vi "3Dplotter.vi"(11 "vectorFile1":path) -> ()   [LabVIEW 2022 SP3]
uses:
  3-Dobject.ctl
  Anemometry/Utilities/EnQMH/EnQcmd.ctl
  <vilib>/Analysis/Matrix/Datatypes/RealMatrix.ctl
  3DplotterData.ctl
  vectorDef.ctl
  coordSys.ctl
  <vilib>/Utility/miscctls.llb/LVRGBAColorTypeDef.ctl
  <vilib>/Utility/miscctls.llb/LV3DPointTypeDef.ctl
  <vilib>/Analysis/baseanly.llb/Real A x B.vi
  <vilib>/Analysis/baseanly.llb/Real Dot Product.vi
  6d968bff-314f-d647-9bf6-e40cfc3952a7.vi
  08ae1a81-02f0-e744-b827-f8e6f0f1c480.vi
  4d4a6871-819a-da47-9cf5-1746fbad62e0.vi
  676242ff-a6cf-3e4f-a0ed-2fc44f2a90a5.vi
  <vilib>/Utility/error.llb/Trim Whitespace One-Sided.vi
  Anemometry/Utilities/EnQMH/EnQmsg.vi
  Anemometry/Utilities/EnQMH/EnQmsgs.vi
  <vilib>/Analysis/baseanly.llb/Real Inverse Matrix.vi
  <vilib>/picture/3D Picture Control/Object/Create Object (name).vi
  <vilib>/picture/3D Picture Control/Object/Add Object (reference).vi
  <vilib>/Comparison/Less/Less Functor/Less Functor.lvclass
  <vilib>/picture/3D Picture Control/Helpers/Apply Texture (no reference).vi
  <vilib>/picture/3D Picture Control/NI_3D Picture Control.lvlib
  <vilib>/Analysis/NI_AALBase.lvlib
  <vilib>/Analysis/Matrix/NI_Matrix.lvlib
panel:
  in  "Tab Control":T1(tab)
  in  "view":i32(slide) min=-1 max=1 step=1
  in  "exportSetup":bool
  in  "importSetup":bool
  in  "Wind Direction Selector":string(combo)
  in  "vectorFile2":path
  in  "Vector Scale":dbl(slide)=100.0 scale=0.2..200.0
  out "Color Ramp":dbl(ramp)
  in  "geometryScale":dbl(slide)=1.0 min=0.1 max=50.0 step=1.0 scale=0.1..50.0 scale format="%#_3g"
  in  "geometry":T2[](array[typedef])
  in  "geometrydZ":dbl(slide) scale=-20.0..20.0
  in  "rampOverride":bool
  in  "rampMax":dbl
  in  "rampMin":dbl
  in  "colourRampClip":dbl min=0.0 max=10.0 step=0.1 format="%#_g%%"
  in  "windrosePath":path
  in  "windrosedXdYdZ":cluster{"dX":dbl, "dY":dbl, "dZ":dbl}
  in  "Apply Mode":T3(ring)=enum."With Modulation"
  in  "windroseScale":dbl(slide)=1.046728971962617 scale=0.5..2.0
  in  "axesColour":u32(colorbox)=16739840
  in  "axes":bool=TRUE
  out "degSymbol":string
  out "eventLoop":errorcluster
  out "stopDolly":bool
  out "actionLoop":errorcluster
  in  "clearVectors":bool
  out "3D Picture":refnum<vi>(3d-picture)
  out "camStandoff":dbl caption="Camera Distance" format="%#.0f"
  in  "camLocn":dbl[](array[numeric]) caption="Camera Location" format="%#.0f"
  in  "Stop":bool
  in  "depthClipping":cluster{sgl, sgl, sgl}(slide)={0.001, 10.0, 9.712047e-08} scale=10.0..0.001 scale format="%.0pm"
  in  "FoV":sgl(slide)=50.0 min=4 max=110 scale=80.0..4.0 scale format="%dº"
  in  "drive":sgl(slide) min=-0.05 max=0.05 scale=0.03..-0.03 scale format="%#.1f"
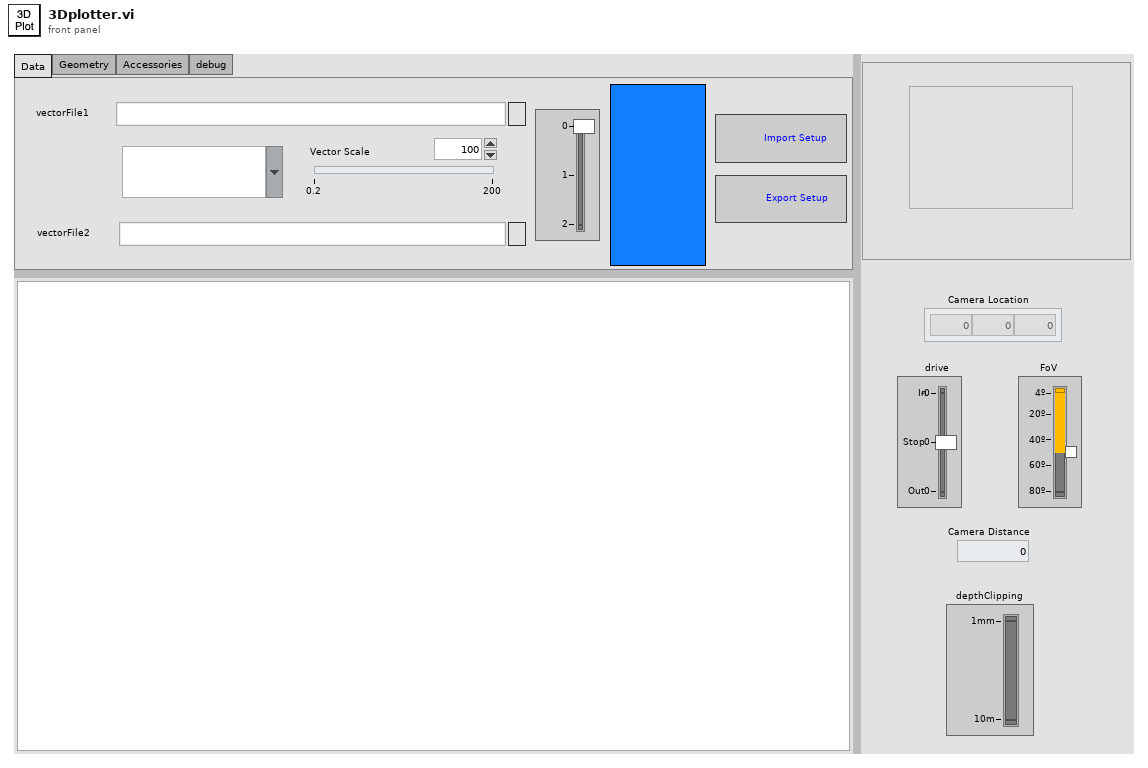
[diagram p1: front panel]
types:
  T1 = enum32{"Data", "Geometry", "Accessories", "debug"}
  T2 = typedef "3-Dobject.ctl" = cluster{"name":string, "path":path, "Colour":u32, "Visible":bool, "dZ":dbl}
  T3 = enum16{"As a Decal", "With Modulation", "With Blending", "As a replacement"}
  T4 = typedef "EnQcmd.ctl" = cluster{"message":string, "payload":variant}
  T5 = typedef "3DplotterData.ctl" = cluster{"mode":bool, "refWorld":refnum<vi>, "refAxes":refnum<vi>, "refWindrose":refnum<vi>, "refGeometry":refnum<vi>, "geometryRefs":refnum<vi>[], "refVectors":refnum<vi>, "refVecs1":refnum<vi>, "refVecs2":refnum<vi>, "vector1Info":T6, "file1scalar":dbl[], "vector2Info":T6, "file2scalar":dbl[], "colourRampVals":cluster{"value":dbl, "colour":u32}[]}
  T6 = typedef "vectorDef.ctl" = cluster{"pointID":string[], "XYZ-WD":dbl[][], "UVW-TI":dbl[][], "CoordSys":T7[]}
  T7 = typedef "coordSys.ctl" = enum16{"Tunnel", "Model"}
  T8 = enum16{"Inherit Value", "No Culling", "Cull Back Face", "Cull Front Face", "Cull Both Faces"}
  T9 = typedef "LVRGBAColorTypeDef.ctl" = cluster{"Red":sgl, "Green":sgl, "Blue":sgl, "Alpha":sgl}
  T10 = enum16{"Inherit Value", "Points", "Wireframe", "Polygons"}
  T11 = enum16{"Normal Bin", "Opaque Bin", "Transparent Bin"}
  T12 = typedef "imagedata.ctl" = cluster{"image type":i32, "image depth":i32, "image":u8[], "mask":u8[], "colors":u32[], "Rectangle":cluster{"left":i16, "top":i16, "right":i16, "bottom":i16}}
  T13 = typedef "Triangle.ctl" = cluster{"V0":sgl[], "V1":sgl[], "V2":sgl[], "E0":sgl[], "E1":sgl[], "E2":sgl[], "n^":sgl[], "nE0^":sgl[], "nE1^":sgl[], "nE2^":sgl[]}
  T14 = typedef "LV3DPointTypeDef.ctl" = cluster{"X":sgl, "Y":sgl, "Z":sgl}
  T15 = typedef "NI_Matrix.lvlib/RealMatrix.ctl" = dbl[][]
  T16 = enum32{"General", "Positive Definite", "Lower Triangular", "Upper Triangular"}
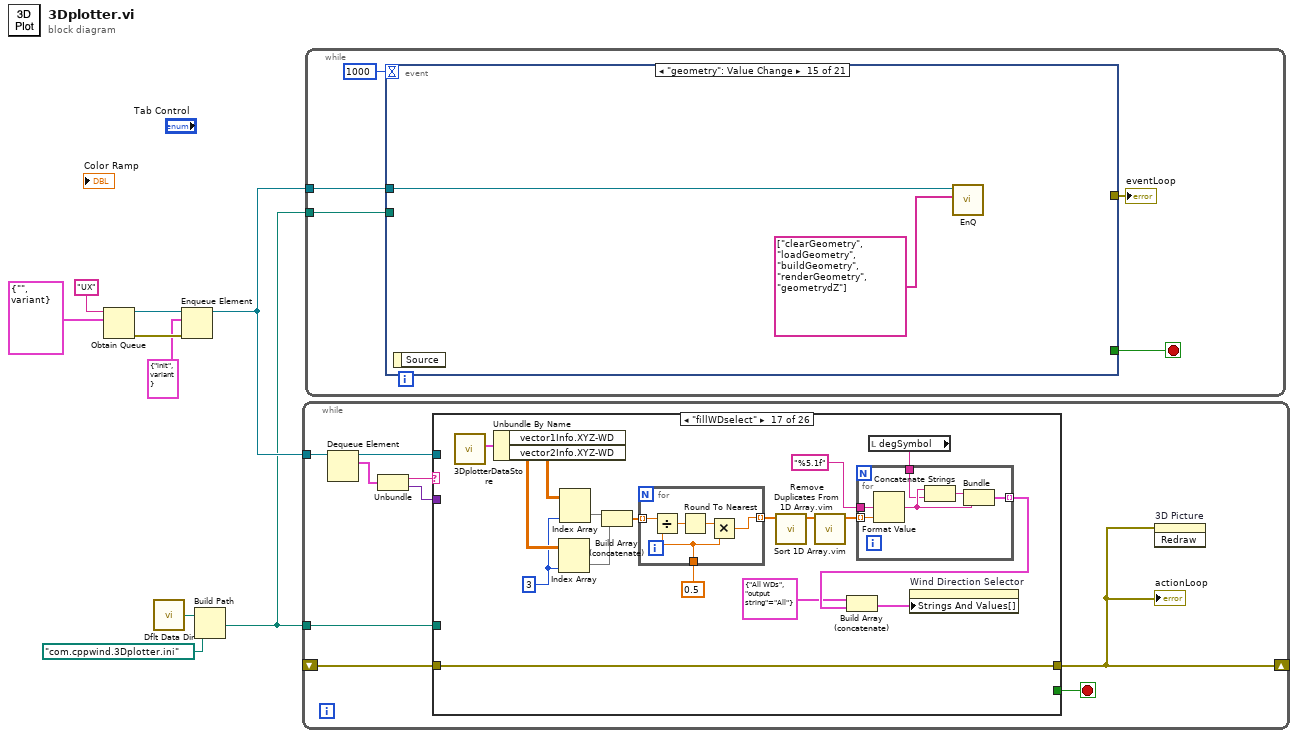
[diagram p0: block diagram]
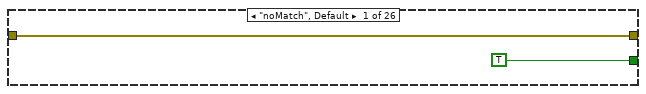
[diagram p2: hidden frame]
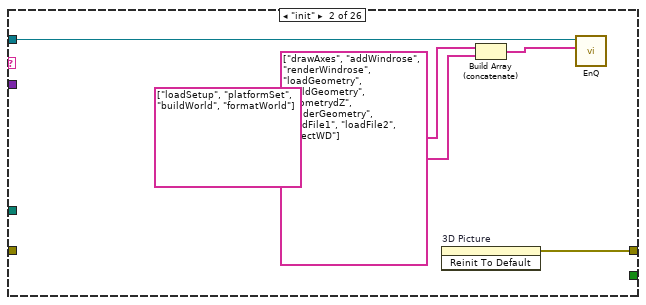
[diagram p3: hidden frame]
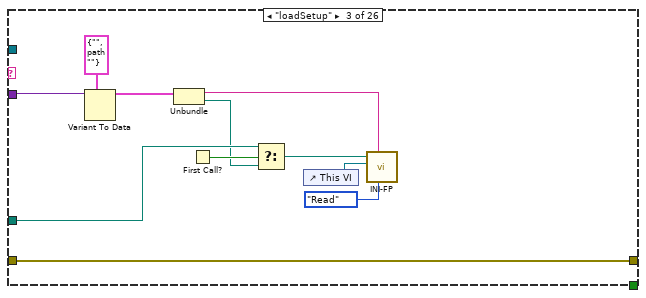
[diagram p4: hidden frame]
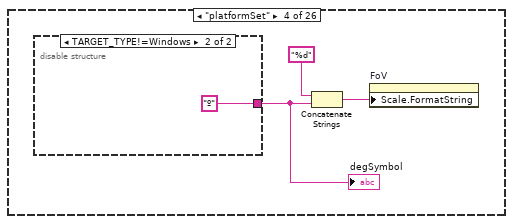
[diagram p5: hidden frame]
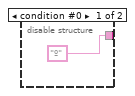
[diagram p6: hidden frame]
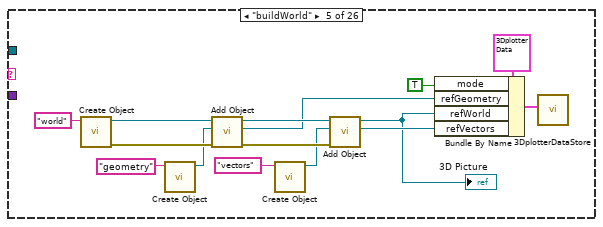
[diagram p7: hidden frame]
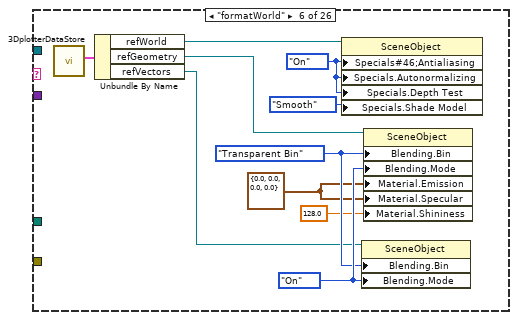
[diagram p8: hidden frame]
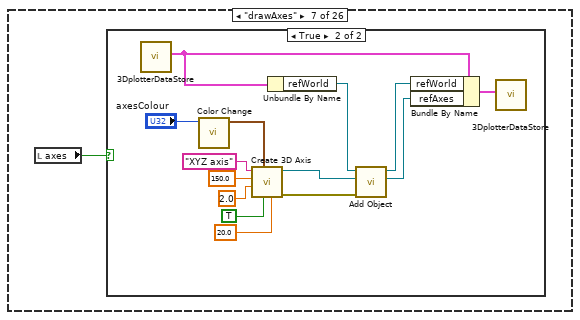
[diagram p9: hidden frame]
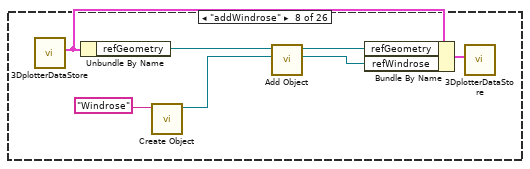
[diagram p11: hidden frame]
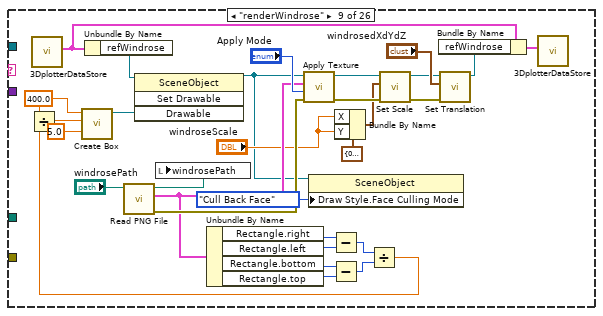
[diagram p12: hidden frame]
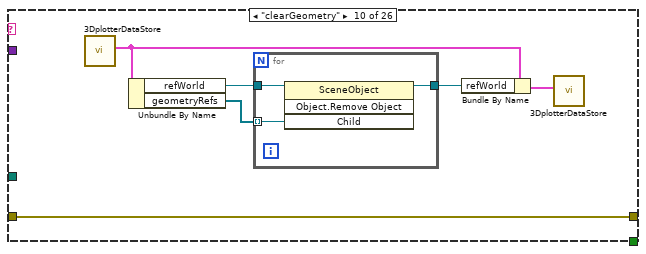
[diagram p13: hidden frame]
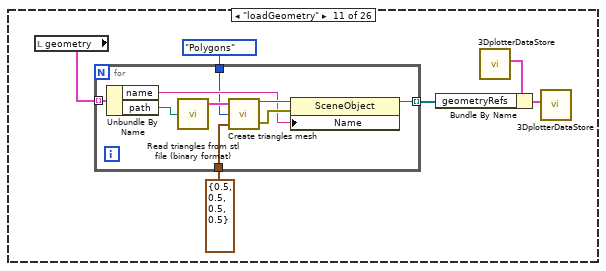
[diagram p14: hidden frame]
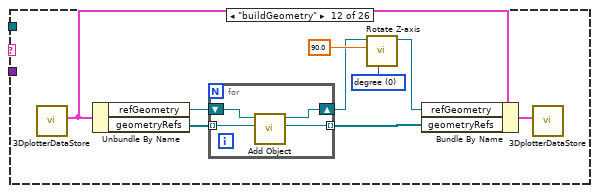
[diagram p15: hidden frame]
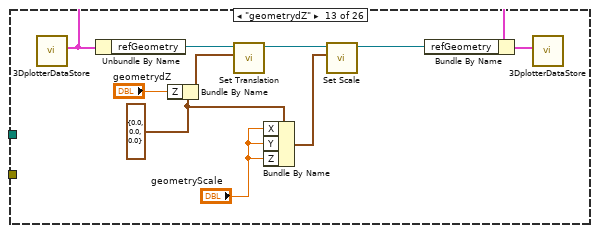
[diagram p16: hidden frame]
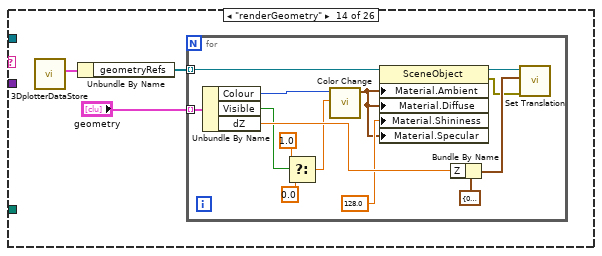
[diagram p17: hidden frame]
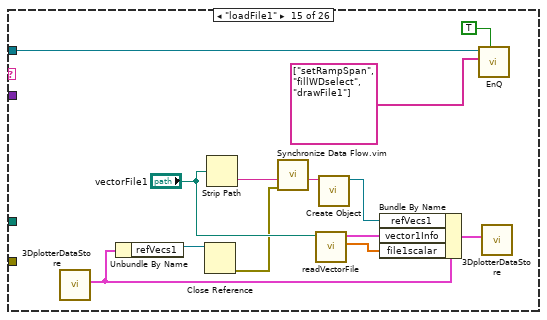
[diagram p18: hidden frame]
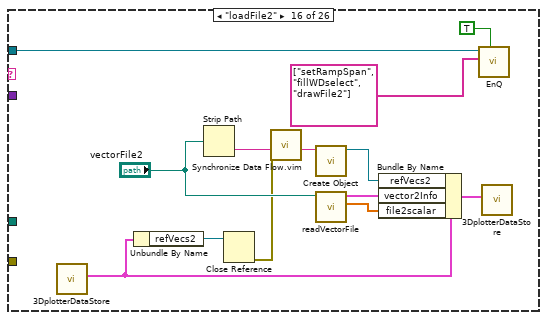
[diagram p19: hidden frame]
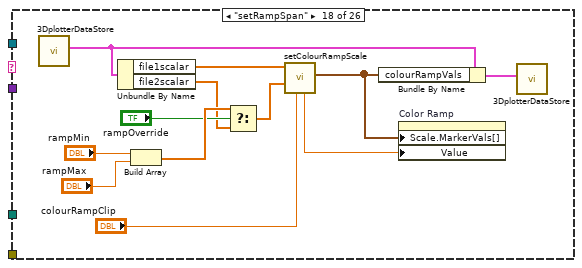
[diagram p20: hidden frame]
diagram:
  n1 = Obtain Queue(name (unnamed)="UX", element data type=T4 {"message"="", "payload"=variant} ("command")) -> (queue out=w5:refnum<queue>, error out=w9:errorcluster)  [unwired: 3 in, 1 out]
  n2 = call <vilib>:"Dflt Data Dir.vi"() -> ("App:Default Data Directory"=w3:path)
  n3 = Enqueue Element(queue=w5, element=T4 {"message"="init", "payload"=variant}, error in (no error)=w9) -> (queue out=w4:refnum<queue>)  [unwired: 1 in, 2 out]
  n4 = Build Path(base path=w3, name or relative path=path "com.cppwind.3Dplotter.ini") -> (appended path=w1:path)
  n5 = while {
    tunnel: w4 -> [w18]
    shift-right: [w10] -> _
    shift-left: _ -> [w13]
    tunnel: w1 -> [w11]
    stop <- w15 stop-if-true
    n6 = Dequeue Element(queue=w18) -> (queue out=w14:refnum<queue>, element=w17:T4)  [unwired: 2 in, 2 out]
    n7 = Unbundle(w17) -> ("message"=w12:string, "payload"=w16:variant)
    n8 = case shown="\"fillWDselect\"" w12 {
      tunnel: w16 -> [_ _ w31 _ _ _ _ _ _ _ _ _ _ _ _ _ _ _ _ _ _ _ _ _ w332 _]
      tunnel: [TRUE _ _ _ _ _ _ _ _ _ _ _ _ _ _ _ _ _ _ _ _ _ _ _ _ TRUE] -> w15
      tunnel: w14 -> [_ w24 _ _ _ _ _ _ _ _ _ _ _ _ w192 w205 _ _ _ _ _ _ _ _ _ _]
      tunnel: [w19 w25 w36 _ _ _ _ _ _ w124 _ _ _ _ _ _ w225 _ _ _ _ _ _ _ w327 _] -> w10
      tunnel: w13 -> [w19 _ w36 _ _ _ _ _ _ w124 _ _ _ _ _ _ w225 _ _ _ _ _ _ _ _ _]
      tunnel: w11 -> [_ _ w28 _ _ _ _ _ _ _ _ _ _ _ _ _ _ _ _ _ _ _ _ _ _ _]
      frame "noMatch", Default {
      }
      frame "init" {
        n9 = invoke on="3D Picture" class="SceneGraphDisp (strict)" method="Reinit To Default"() -> (error out=w25:errorcluster)  [unwired: 3 in, 2 out]
        n10 = Build Array (concatenate)(string[] ["loadSetup", "platformSet", "buildWorld", "formatWorld"] ("messages"), string[] ["drawAxes", "addWindrose", "renderWindrose", "loadGeometry", "buildGeometry", "geometrydZ", "renderGeometry", "loadFile1", "loadFile2", "selectWD"] ("messages")) -> (w21:string[])
        n11 = call-poly "EnQ.vi"("messages"=w21, "EnQin"=w24) -> ()  [unwired: 7 in, 3 out]
      }
      frame "loadSetup" {
        n12 = Variant To Data(type=cluster{string, "appended path":path} {"", "appended path"=path ""} ("output cluster"), Variant=w31) -> (data=w33:cluster{string, "appended path":path})  [unwired: 1 in, 1 out]
        n13 = Unbundle(w33) -> (w30:string, "appended path"=w27:path)
        n14 = First Call?() -> (First Call?: T/F=w29:bool)
        n15 = Select(t=w28, s=w29, f=w27) -> (s? t:f=w26:path)
        n16 = control-ref of="This VI"() -> (w35:refnum<vi>)
        n17 = call "INI-FP.vi"("Mode"=enum16{"Read", "Write"}."Read", "prompt"=w30, "VIreference"=w35, "INIfilepathIn"=w26) -> ()  [unwired: 6 in, 2 out]
      }
      frame "platformSet" {
        n18 = disable-structure shown="TARGET_TYPE!=Windows" {
          disable-tunnel: ["º" ("Scale.Format String") "º" ("Scale.Format String")] -> w37
          frame condition #0 {
          }
          frame condition #1 (active) {
          }
        }
        "degSymbol" <- w37
        n19 = Concatenate Strings("%d" ("Scale.Format String"), w37) -> (w39:string)
        n20 = property on="FoV" class="Slide (strict)"("Scale.FormatString"=w39) -> ()  [unwired: 2 in, 2 out]
      }
      frame "buildWorld" {
        n21 = call-poly <vilib>:"Create Object.vi"("Name"="world") -> ("error out"=w48:errorcluster, "Scene:New Object"=w50:refnum<vi>)  [unwired: 9 in]
        n22 = call-poly <vilib>:"Create Object.vi"("Name"="geometry") -> ("Scene:New Object"=w44:refnum<vi>)  [unwired: 9 in, 1 out]
        n23 = call-poly <vilib>:"Add Object.vi"("error in (no error)"=w48, "New Object In"=w44, "Scene Object In"=w50) -> ("error out"=w47:errorcluster, "New Object Out"=w46:refnum<vi>, "Scene Object Out"=w49:refnum<vi>)  [unwired: 6 in]
        n24 = call-poly <vilib>:"Create Object.vi"("Name"="vectors") -> ("Scene:New Object"=w43:refnum<vi>)  [unwired: 9 in, 1 out]
        n25 = call-poly <vilib>:"Add Object.vi"("error in (no error)"=w47, "New Object In"=w43, "Scene Object In"=w49) -> ("New Object Out"=w45:refnum<vi>, "Scene Object Out"=w42:refnum<vi>)  [unwired: 6 in, 1 out]
        "3D Picture" <- w42
        n26 = Bundle By Name(cluster=T5 {"mode"=FALSE, "refWorld"=refnum, "refAxes"=refnum, "refWindrose"=refnum, "refGeometry"=refnum, "geometryRefs"=[], "refVectors"=refnum, "refVecs1"=refnum, "refVecs2"=refnum, "vector1Info"={"pointID"=[], "XYZ-WD"=[], "UVW-TI"=[], "CoordSys"=[]}, "file1scalar"=[], "vector2Info"={"pointID"=[], "XYZ-WD"=[], "UVW-TI"=[], "CoordSys"=[]}, "file2scalar"=[], "colourRampVals"=[]} ("3DplotterDataIn"), "mode"=TRUE, "refGeometry"=w46, "refWorld"=w42, "refVectors"=w45) -> (w53:T5)
        n27 = call "3DplotterDataStore.vi"("3DplotterDataIn"=w53) -> ()  [unwired: 10 in, 1 out]
      }
      frame "formatWorld" {
        w62 = enum16{"Inherit Value", "Off", "On"}."On" ("Specials:Anti-aliasing")
        w64 = T9 {"Red"=0.0, "Green"=0.0, "Blue"=0.0, "Alpha"=0.0} ("Material:Emission")
        w66 = enum16{"Inherit Value", "Off", "On"}."On" ("Blending:Mode")
        w65 = T11."Transparent Bin" ("Blending:Bin")
        n28 = call "3DplotterDataStore.vi"() -> ("3DplotterDataOut"=w60:T5)  [unwired: 11 in]
        n29 = Unbundle By Name(w60) -> ("refWorld"=w59:refnum<vi>, "refGeometry"=w58:refnum<vi>, "refVectors"=w57:refnum<vi>)
        n30 = property class="SceneObject"(reference=w59, "Specials#46;Antialiasing"=w62, "Specials.Autonormalizing"=w62, "Specials.Depth Test"=w62, "Specials.Shade Model"=enum16{"Inherit Value", "Flat", "Smooth"}."Smooth" ("Specials:Shade Model")) -> ()  [unwired: 1 in, 2 out]
        n31 = property class="SceneObject"(reference=w57, "Blending.Bin"=w65, "Blending.Mode"=w66) -> ()  [unwired: 1 in, 2 out]
        n32 = property class="SceneObject"(reference=w58, "Blending.Bin"=w65, "Blending.Mode"=w66, "Material.Emission"=w64, "Material.Specular"=w64, "Material.Shininess"=sgl 128.0 ("Material:Shininess")) -> ()  [unwired: 1 in, 2 out]
      }
      frame "drawAxes" {
        n33 = local read "axes"() -> (w67:bool)
        n34 = case shown="True" w67 {
          frame False {
          }
          frame True {
            n35 = call "3DplotterDataStore.vi"() -> ("3DplotterDataOut"=w75:T5)  [unwired: 11 in]
            n36 = call <vilib>:"Color Change.vi"("Color"="axesColour") -> ("RGBA"=w69:cluster{"R":sgl, "G":sgl, "B":sgl, "A":sgl})  [unwired: 10 in]
            n37 = call <vilib>:"Create 3D Axis.vi"("Character Size"=sgl 20.0, "Axis label?"=TRUE, "Color"=w69, "Radius"=sgl 2.0, "Length"=sgl 150.0, "Name"="XYZ axis") -> ("error out"=w71:errorcluster, "New Object Refnum"=w73:refnum<vi>)  [unwired: 4 in]
            n38 = Unbundle By Name(w75) -> ("refWorld"=w74:refnum<vi>)
            n39 = call-poly <vilib>:"Add Object.vi"("error in (no error)"=w71, "New Object In"=w73, "Scene Object In"=w74) -> ("New Object Out"=w72:refnum<vi>, "Scene Object Out"=w70:refnum<vi>)  [unwired: 6 in, 1 out]
            n40 = Bundle By Name(cluster=w75, "refWorld"=w70, "refAxes"=w72) -> (w81:T5)
            n41 = call "3DplotterDataStore.vi"("3DplotterDataIn"=w81) -> ()  [unwired: 10 in, 1 out]
          }
        }
      }
      frame "addWindrose" {
        n42 = call "3DplotterDataStore.vi"() -> ("3DplotterDataOut"=w85:T5)  [unwired: 11 in]
        n43 = Unbundle By Name(w85) -> ("refGeometry"=w88:refnum<vi>)
        n44 = call-poly <vilib>:"Create Object.vi"("Name"="Windrose") -> ("Scene:New Object"=w82:refnum<vi>)  [unwired: 9 in, 1 out]
        n45 = call-poly <vilib>:"Add Object.vi"("New Object In"=w82, "Scene Object In"=w88) -> ("New Object Out"=w83:refnum<vi>, "Scene Object Out"=w84:refnum<vi>)  [unwired: 7 in, 1 out]
        n46 = Bundle By Name(cluster=w85, "refGeometry"=w84, "refWindrose"=w83) -> (w86:T5)
        n47 = call "3DplotterDataStore.vi"("3DplotterDataIn"=w86) -> ()  [unwired: 10 in, 1 out]
      }
      frame "renderWindrose" {
        w100 = sgl 400.0 ("Length X")
        n48 = call "3DplotterDataStore.vi"() -> ("3DplotterDataOut"=w112:T5)  [unwired: 11 in]
        n49 = Unbundle By Name(w112) -> ("refWindrose"=w111:refnum<vi>)
        n50 = call <vilib>:"Read PNG File.vi"("path to PNG file"="windrosePath") -> ("error out"=w116:errorcluster, "image data"=w109:T12, "path"=w89:path)  [unwired: 8 in]
        n51 = local write "windrosePath"(w89) -> ()
        n52 = Unbundle By Name(w109) -> ("Rectangle.right"=w108:i16, "Rectangle.left"=w107:i16, "Rectangle.bottom"=w106:i16, "Rectangle.top"=w105:i16)
        n53 = Subtract(x=w108, y=w107) -> (x-y=w104:i16)
        n54 = Subtract(x=w106, y=w105) -> (x-y=w103:i16)
        n55 = Bundle By Name(cluster=cluster{"X":sgl, "Y":sgl, "Z":sgl} {"X"=0.0, "Y"=0.0, "Z"=0.0} ("Scale"), "X"="windroseScale", "Y"="windroseScale") -> (w94:cluster{"X":sgl, "Y":sgl, "Z":sgl})
        n56 = Divide(x=w104, y=w103) -> (x/y=w102:dbl)
        n57 = Divide(x=w100, y=w102) -> (x/y=w101:dbl)
        n58 = call <vilib>:"Create Box.vi"("Length Z"=sgl 5.0, "Length Y"=w101, "Length X"=w100) -> ("New Box Refnum"=w110:refnum<vi>)  [unwired: 7 in, 1 out]
        n59 = invoke class="SceneObject" method="Set Drawable"(reference=w111, "Drawable"=w110) -> (reference out=w91:refnum<vi>)  [unwired: 2 in, 3 out]
        n60 = call-poly <vilib>:"Apply Texture.vi"("error in (no error)"=w116, "Apply Mode"="Apply Mode", "Image Data"=w109, "Scene Object In"=w91) -> ("error out"=w98:errorcluster, "Scene Object Out"=w99:refnum<vi>)  [unwired: 6 in]
        n61 = property class="SceneObject"(reference=w91, "Draw Style.Face Culling Mode"=T8."Cull Back Face" ("Draw Style:Face Culling Mode")) -> ()  [unwired: 1 in, 2 out]
        n62 = call <vilib>:"Set Scale.vi"("error in (no error)"=w98, "Scale"=w94, "Scene Object"=w99) -> ("error out"=w96:errorcluster, "Scaled Object"=w97:refnum<vi>)  [unwired: 7 in]
        n63 = call <vilib>:"Set Translation.vi"("error in (no error)"=w96, "Translation"="windrosedXdYdZ", "Scene Object"=w97) -> ("Translated Object"=w92:refnum<vi>)  [unwired: 7 in, 1 out]
        n64 = Bundle By Name(cluster=w112, "refWindrose"=w92) -> (w113:T5)
        n65 = call "3DplotterDataStore.vi"("3DplotterDataIn"=w113) -> ()  [unwired: 10 in, 1 out]
      }
      frame "clearGeometry" {
        n66 = call "3DplotterDataStore.vi"() -> ("3DplotterDataOut"=w122:T5)  [unwired: 11 in]
        n67 = Unbundle By Name(w122) -> ("refWorld"=w121:refnum<vi>, "geometryRefs"=w120:refnum<vi>[])
        n68 = for {
          tunnel: w121 -> [w127]
          tunnel: w120 -> [w126] mode=indexing
          tunnel: [w125] -> w119
          n69 = invoke class="SceneObject" method="Object.Remove Object"(reference=w127, "Child"=w126) -> (reference out=w125:refnum<vi>)  [unwired: 2 in, 3 out]
        }
        n70 = Bundle By Name(cluster=w122, "refWorld"=w119) -> (w123:T5)
        n71 = call "3DplotterDataStore.vi"("3DplotterDataIn"=w123) -> ()  [unwired: 10 in, 1 out]
      }
      frame "loadGeometry" {
        n72 = local read "geometry"() -> (w133:T2[])
        n73 = for {
          tunnel: w133 -> [w142] mode=indexing
          tunnel: [w136] -> w130 mode=indexing
          tunnel: T10."Polygons" ("Render mode") -> [w135]
          tunnel: T9 {"Red"=0.5, "Green"=0.5, "Blue"=0.5, "Alpha"=0.5} ("Colour") -> [w134]
          n74 = Unbundle By Name(w142) -> ("name"=w137:string, "path"=w140:path)
          n75 = call "Read triangles from stl file (binary format).vi"("STL file path"=w140) -> ("Triangles array"=w141:T13[])  [unwired: 2 out]
          n76 = call "Create triangles mesh.vi"("Colour"=w134, "Render mode"=w135, "Triangles array"=w141) -> ("Error out"=w138:errorcluster, "Triangle mesh out"=w139:refnum<vi>)
          n77 = property class="SceneObject"(reference=w139, error in=w138, "Name"=w137) -> (reference out=w136:refnum<vi>)  [unwired: 1 out]
        }
        n78 = call "3DplotterDataStore.vi"() -> ("3DplotterDataOut"=w131:T5)  [unwired: 11 in]
        n79 = Bundle By Name(cluster=w131, "geometryRefs"=w130) -> (w132:T5)
        n80 = call "3DplotterDataStore.vi"("3DplotterDataIn"=w132) -> ()  [unwired: 10 in, 1 out]
      }
      frame "buildGeometry" {
        w146 = u16 0 items=["degree", "radians"] ("angle unit")
        n81 = call "3DplotterDataStore.vi"() -> ("3DplotterDataOut"=w149:T5)  [unwired: 11 in]
        n82 = Unbundle By Name(w149) -> ("refGeometry"=w151:refnum<vi>, "geometryRefs"=w150:refnum<vi>[])
        n83 = for {
          shift-right: [w154] -> w144
          shift-left: w151 -> [w155]
          tunnel: w150 -> [w153] mode=indexing
          tunnel: [w152] -> w148 mode=indexing
          n84 = call-poly <vilib>:"Add Object.vi"("New Object In"=w153, "Scene Object In"=w155) -> ("New Object Out"=w152:refnum<vi>, "Scene Object Out"=w154:refnum<vi>)  [unwired: 7 in, 1 out]
        }
        n85 = call <vilib>:"Rotate Z-axis.vi"("angle unit"=w146, "angle"=sgl 90.0, "Scene Object In"=w144) -> ("Scene Object Out"=w143:refnum<vi>)  [unwired: 7 in, 1 out]
        n86 = Bundle By Name(cluster=w149, "refGeometry"=w143, "geometryRefs"=w148) -> (w147:T5)
        n87 = call "3DplotterDataStore.vi"("3DplotterDataIn"=w147) -> ()  [unwired: 10 in, 1 out]
      }
      frame "geometrydZ" {
        w158 = cluster{"X":sgl, "Y":sgl, "Z":sgl} {"X"=0.0, "Y"=0.0, "Z"=0.0} ("Translation")
        n88 = call "3DplotterDataStore.vi"() -> ("3DplotterDataOut"=w165:T5)  [unwired: 11 in]
        n89 = Unbundle By Name(w165) -> ("refGeometry"=w163:refnum<vi>)
        n90 = Bundle By Name(cluster=w158, "Z"="geometrydZ") -> (w161:cluster{"X":sgl, "Y":sgl, "Z":sgl})
        n91 = call <vilib>:"Set Translation.vi"("Translation"=w161, "Scene Object"=w163) -> ("Translated Object"=w162:refnum<vi>)  [unwired: 8 in, 1 out]
        n92 = Bundle By Name(cluster=w158, "X"="geometryScale", "Y"="geometryScale", "Z"="geometryScale") -> (w157:cluster{"X":sgl, "Y":sgl, "Z":sgl})
        n93 = call <vilib>:"Set Scale.vi"("Scale"=w157, "Scene Object"=w162) -> ("Scaled Object"=w159:refnum<vi>)  [unwired: 8 in, 1 out]
        n94 = Bundle By Name(cluster=w165, "refGeometry"=w159) -> (w164:T5)
        n95 = call "3DplotterDataStore.vi"("3DplotterDataIn"=w164) -> ()  [unwired: 10 in, 1 out]
      }
      frame "renderGeometry" {
        n96 = call "3DplotterDataStore.vi"() -> ("3DplotterDataOut"=w168:T5)  [unwired: 11 in]
        n97 = Unbundle By Name(w168) -> ("geometryRefs"=w167:refnum<vi>[])
        n98 = for {
          tunnel: "geometry" -> [w182] mode=indexing
          tunnel: w167 -> [w178] mode=indexing
          n99 = Unbundle By Name(w182) -> ("Colour"=w177:u32, "Visible"=w173:bool, "dZ"=w180:dbl)
          n100 = Select(t=1.0, s=w173, f=0.0) -> (s? t:f=w172:dbl)
          n101 = call <vilib>:"Color Change.vi"("Alpha"=w172, "Color"=w177) -> ("RGBA"=w169:cluster{"R":sgl, "G":sgl, "B":sgl, "A":sgl})  [unwired: 9 in]
          n102 = property class="SceneObject"(reference=w178, "Material.Ambient"=w169, "Material.Diffuse"=w169, "Material.Shininess"=sgl 128.0 ("Material:Shininess"), "Material.Specular"=w169) -> (reference out=w176:refnum<vi>, error out=w171:errorcluster)  [unwired: 1 in]
          n103 = Bundle By Name(cluster=cluster{"X":sgl, "Y":sgl, "Z":sgl} {"X"=0.0, "Y"=0.0, "Z"=0.0} ("Translation"), "Z"=w180) -> (w179:cluster{"X":sgl, "Y":sgl, "Z":sgl})
          n104 = call <vilib>:"Set Translation.vi"("error in (no error)"=w171, "Translation"=w179, "Scene Object"=w176) -> ()  [unwired: 7 in, 2 out]
        }
      }
      frame "loadFile1" {
        n105 = call "3DplotterDataStore.vi"() -> ("3DplotterDataOut"=w187:T5)  [unwired: 11 in]
        n106 = Unbundle By Name(w187) -> ("refVecs1"=w186:refnum<vi>)
        n107 = Close Reference(reference=w186) -> (error out=w184:errorcluster)  [unwired: 1 in]
        n108 = Strip Path(path="vectorFile1") -> (name=w195:string)  [unwired: 1 out]
        n109 = call "Synchronize Data Flow.vim"("input 4"=w184, "input 3"=w195) -> ("output 3"=w185:string)  [unwired: 2 in, 3 out]
        n110 = call "readVectorFile.vi"("vectorFile"="vectorFile1") -> ("scalar"=w193:dbl[], "vectorInfo"=w191:T6)  [unwired: 9 in]
        n111 = call-poly <vilib>:"Create Object.vi"("Name"=w185) -> ("Scene:New Object"=w190:refnum<vi>)  [unwired: 9 in, 1 out]
        n112 = Bundle By Name(cluster=w187, "refVecs1"=w190, "vector1Info"=w191, "file1scalar"=w193) -> (w194:T5)
        n113 = call-poly "EnQ.vi"("priority?"=TRUE, "messages"=string[] ["setRampSpan", "fillWDselect", "drawFile1"], "EnQin"=w192) -> ()  [unwired: 6 in, 3 out]
        n114 = call "3DplotterDataStore.vi"("3DplotterDataIn"=w194) -> ()  [unwired: 10 in, 1 out]
      }
      frame "loadFile2" {
        n115 = call "3DplotterDataStore.vi"() -> ("3DplotterDataOut"=w200:T5)  [unwired: 11 in]
        n116 = Unbundle By Name(w200) -> ("refVecs2"=w199:refnum<vi>)
        n117 = Strip Path(path="vectorFile2") -> (name=w208:string)  [unwired: 1 out]
        n118 = Close Reference(reference=w199) -> (error out=w197:errorcluster)  [unwired: 1 in]
        n119 = call "Synchronize Data Flow.vim"("input 4"=w197, "input 3"=w208) -> ("output 3"=w198:string)  [unwired: 2 in, 3 out]
        n120 = call-poly <vilib>:"Create Object.vi"("Name"=w198) -> ("Scene:New Object"=w203:refnum<vi>)  [unwired: 9 in, 1 out]
        n121 = call "readVectorFile.vi"("vectorFile"="vectorFile2") -> ("scalar"=w206:dbl[], "vectorInfo"=w204:T6)  [unwired: 9 in]
        n122 = Bundle By Name(cluster=w200, "refVecs2"=w203, "vector2Info"=w204, "file2scalar"=w206) -> (w207:T5)
        n123 = call-poly "EnQ.vi"("priority?"=TRUE, "messages"=string[] ["setRampSpan", "fillWDselect", "drawFile2"], "EnQin"=w205) -> ()  [unwired: 6 in, 3 out]
        n124 = call "3DplotterDataStore.vi"("3DplotterDataIn"=w207) -> ()  [unwired: 10 in, 1 out]
      }
      frame "fillWDselect" {
        w218 = 3 ("disabled index (col)")
        n125 = call "3DplotterDataStore.vi"() -> ("3DplotterDataOut"=w224:T5)  [unwired: 11 in]
        n126 = Unbundle By Name(w224) -> ("vector1Info.XYZ-WD"=w223:dbl[][], "vector2Info.XYZ-WD"=w219:dbl[][])
        n127 = Index Array(array=w219, index (col)=w218) -> (element=w217:dbl[])  [unwired: 1 in]
        n128 = Index Array(array=w223, index (col)=w218) -> (element=w222:dbl[])  [unwired: 1 in]
        n129 = Build Array (concatenate)(w222, w217) -> (w212:dbl[])
        n130 = for {
          tunnel: w212 -> [w228] mode=indexing
          tunnel: 0.5 -> [w227]
          tunnel: [w226] -> w211 mode=indexing
          n131 = Divide(x=w228, y=w227) -> (x/y=w229:dbl)
          n132 = Round To Nearest(number=w229) -> (nearest integer value=w230:dbl)
          n133 = Multiply(x=w230, y=w227) -> (x*y=w226:dbl)
        }
        n134 = call "Remove Duplicates From 1D Array.vim"("array"=w211) -> ("array with duplicates removed"=w221:dbl[])  [unwired: 10 in]
        n135 = call "Sort 1D Array.vim"("unsorted array"=w221) -> ("sorted array"=w213:dbl[])  [unwired: 10 in]
        n136 = local read "degSymbol"() -> (w209:string)
        n137 = for {
          tunnel: w213 -> [w236] mode=indexing
          tunnel: "%5.1f" ("format string") -> [w235]
          tunnel: [w232] -> w216 mode=indexing
          tunnel: w209 -> [w231]
          n138 = Format Value(format string=w235, value (0)=w236) -> (output string=w233:string)  [unwired: 1 in]
          n139 = Concatenate Strings(w233, w231) -> (w234:string)
          n140 = Bundle(w234, "output string"=w233) -> (w232:cluster{string, "output string":string})  [unwired: 1 in]
        }
        n141 = Build Array (concatenate)(cluster{string, "output string":string} {"All WDs", "output string"="All"}, w216) -> (w214:cluster{string, "output string":string}[])
        n142 = property on="Wind Direction Selector" class="CmbBox"("Strings And Values[]"=w214) -> ()  [unwired: 2 in, 2 out]
      }
      frame "setRampSpan" {
        n143 = call "3DplotterDataStore.vi"() -> ("3DplotterDataOut"=w247:T5)  [unwired: 11 in]
        n144 = Unbundle By Name(w247) -> ("file1scalar"=w246:dbl[], "file2scalar"=w238:dbl[])
        n145 = Build Array("rampMin", "rampMax") -> (w240:dbl[])
        n146 = Select(t=w240, s="rampOverride", f=w238) -> (s? t:f=w237:dbl[])
        n147 = call "setColourRampScale.vi"("scaleClipPercentile"="colourRampClip", "comaparativeData"=w237, "baselineData"=w246) -> ("colourRampVals"=w245:cluster{"value":dbl, "colour":u32}[], "whitePoint"=w244:dbl)  [unwired: 7 in]
        n148 = Bundle By Name(cluster=w247, "colourRampVals"=w245) -> (w248:T5)
        n149 = property on="Color Ramp" class="ColRmp (strict)"("Scale.MarkerVals[]"=w245, "Value"=w244) -> ()  [unwired: 2 in, 2 out]
        n150 = call "3DplotterDataStore.vi"("3DplotterDataIn"=w248) -> ()  [unwired: 10 in, 1 out]
      }
      frame "drawFile1" {
        n151 = call "3DplotterDataStore.vi"() -> ("3DplotterDataOut"=w252:T5)  [unwired: 11 in]
        n152 = Unbundle By Name(w252) -> ("refVectors"=w254:refnum<vi>, "vector1Info"=w260:T6, "refVecs1"=w256:refnum<vi>, "colourRampVals"=w255:cluster{"value":dbl, "colour":u32}[])
        n153 = local read "Vector Scale"() -> (w258:dbl)
        n154 = call "vectorField.vi"("mostCoords"=coordSys."Model", "thiccness"=sgl 5.0, "colourRampVals"=w255, "scale"=w258, "style"=enum16{"Round", "Square"}."Round", "vectorInfo"=w260, "SceneObject in"=w256) -> ("SceneObject out"=w257:refnum<vi>)  [unwired: 3 in, 1 out]
        n155 = call-poly <vilib>:"Add Object.vi"("New Object In"=w257, "Scene Object In"=w254) -> ("New Object Out"=w251:refnum<vi>, "Scene Object Out"=w250:refnum<vi>)  [unwired: 7 in, 1 out]
        n156 = Bundle By Name(cluster=w252, "refVectors"=w250, "refVecs1"=w251) -> (w253:T5)
        n157 = call "3DplotterDataStore.vi"("3DplotterDataIn"=w253) -> ()  [unwired: 10 in, 1 out]
      }
      frame "drawFile2" {
        n158 = call "3DplotterDataStore.vi"() -> ("3DplotterDataOut"=w265:T5)  [unwired: 11 in]
        n159 = Unbundle By Name(w265) -> ("refVectors"=w270:refnum<vi>, "vector2Info"=w273:T6, "refVecs2"=w268:refnum<vi>, "colourRampVals"=w267:cluster{"value":dbl, "colour":u32}[])
        n160 = local read "Vector Scale"() -> (w271:dbl)
        n161 = call "vectorField.vi"("mostCoords"=coordSys."Model", "thiccness"=sgl 5.0, "colourRampVals"=w267, "scale"=w271, "style"=enum16{"Round", "Square"}."Square", "vectorInfo"=w273, "SceneObject in"=w268) -> ("SceneObject out"=w269:refnum<vi>)  [unwired: 3 in, 1 out]
        n162 = call-poly <vilib>:"Add Object.vi"("New Object In"=w269, "Scene Object In"=w270) -> ("New Object Out"=w263:refnum<vi>, "Scene Object Out"=w264:refnum<vi>)  [unwired: 7 in, 1 out]
        n163 = Bundle By Name(cluster=w265, "refVectors"=w264, "refVecs2"=w263) -> (w266:T5)
        n164 = call "3DplotterDataStore.vi"("3DplotterDataIn"=w266) -> ()  [unwired: 10 in, 1 out]
      }
      frame "selectWD" {
        n165 = call "3DplotterDataStore.vi"() -> ("3DplotterDataOut"=w284:T5)  [unwired: 11 in]
        n166 = call <vilib>:"Trim Whitespace.vi"("string"="Wind Direction Selector") -> ("trimmed string"=w279:string)  [unwired: 1 in]
        n167 = Unbundle By Name(w284) -> ("refVecs1"=w285:refnum<vi>, "refVecs2"=w280:refnum<vi>)
        n168 = case shown="1, Default" "view" {
          tunnel: [TRUE ("visible? (T)") w288 FALSE ("visible? (T)")] -> w276
          tunnel: [FALSE ("visible? (T)") w288 TRUE ("visible? (T)")] -> w275
          frame 0 {
          }
          frame 1, Default {
            w288 = TRUE ("visible? (T)")
          }
          frame 2 {
          }
        }
        n169 = Match Pattern(string="Wind Direction Selector", regular expression="All") -> (offset past match=w281:i32)  [unwired: 1 in, 3 out]
        n170 = Greater Or Equal To 0?(x=w281) -> (x >= 0?=w278:bool)
        n171 = call "showOrHideByName.vi"("showAll (F)"=w278, "visible? (T)"=w275, "matchString"=w279, "SceneObject in"=w280) -> ()  [unwired: 7 in, 1 out]
        n172 = call "showOrHideByName.vi"("showAll (F)"=w278, "visible? (T)"=w276, "matchString"=w279, "SceneObject in"=w285) -> ()  [unwired: 7 in, 1 out]
      }
      frame "clearVectors" {
        n173 = call "3DplotterDataStore.vi"() -> ("3DplotterDataOut"=w296:T5)  [unwired: 11 in]
        n174 = Unbundle By Name(w296) -> ("refVectors"=w293:refnum<vi>, "refVecs1"=w292:refnum<vi>, "refVecs2"=w291:refnum<vi>)
        n175 = Build Array(w292, w291) -> (w295:refnum<vi>[])
        n176 = call "getAllDescendants.vi"("parentsIn"=w295) -> ("allDescendants"=w294:refnum<vi>[])  [unwired: 8 in, 2 out]
        n177 = for {
          tunnel: w293 -> [w299]
          tunnel: w294 -> [w298] mode=indexing
          n178 = invoke class="SceneObject" method="Object.Remove Object"(reference=w299, "Child"=w298) -> (error out=w297:errorcluster)  [unwired: 2 in, 3 out]
          n179 = Close Reference(reference=w298, error in (no error)=w297) -> ()  [unwired: 1 out]
        }
      }
      frame "deleteAxes" {
        n180 = call "3DplotterDataStore.vi"() -> ("3DplotterDataOut"=w303:T5)  [unwired: 11 in]
        n181 = Unbundle By Name(w303) -> ("refWorld"=w301:refnum<vi>, "refAxes"=w302:refnum<vi>)
        n182 = invoke class="SceneObject" method="Object.Remove Object"(reference=w301, "Child"=w302) -> (reference out=w300:refnum<vi>)  [unwired: 2 in, 3 out]
        n183 = Bundle By Name(cluster=w303, "refWorld"=w300) -> (w304:T5)
        n184 = call "3DplotterDataStore.vi"("3DplotterDataIn"=w304) -> ()  [unwired: 10 in, 1 out]
      }
      frame "dollyMove" {
        n185 = while {
          tunnel: [sgl 0.0 ("drive")] -> w305
          stop <- w316 stop-if-true
          w325 = T14 {"X"=0.0, "Y"=0.0, "Z"=1.0} ("Up Direction")
          n186 = local read "camLocn"() -> (w319:dbl[])
          n187 = Increment(x="drive") -> (x+1=w322:sgl)
          n188 = Less Than 0?(x="drive") -> (x < 0?=w313:bool)
          n189 = Greater Than 0?(x="drive") -> (x > 0?=w307:bool)
          n190 = call-poly <vilib>:"Dot Product.vi"("Y Vector"=w319, "X Vector"=w319) -> ("X * Y"=w318:dbl)  [unwired: 1 out]
          n191 = Multiply(x=w322, y=w319) -> (x*y=w320:dbl[])
          n192 = Square Root(x=w318) -> (sqrt(x)=w310:dbl)
          n193 = Wait (ms)(milliseconds to wait=u32 50) -> ()  [unwired: 1 out]
          n194 = Greater?(x=w310, y=10000.0) -> (0:w308:bool)
          n195 = property on="camLocn" class="Arr (strict)"("Val(Sgnl)"=w320) -> ()  [unwired: 2 in, 2 out]
          n196 = Less?(x=w310, y=100.0 ("x")) -> (x < y?=w315:bool)
          n197 = Array To Cluster(array=w320) -> (cluster=w326:cluster{"[0]":dbl, "[1]":dbl, "[2]":dbl})
          n198 = And(x=w315, y=w313) -> (x .and. y?=w314:bool)
          n199 = And(x=w307, y=w308) -> (x .and. y?=w306:bool)
          n200 = invoke on="3D Picture" class="SceneGraphDisp (strict)" method="Setup Camera"("Camera Position"=w326, "Target"=w325, "Up Direction"=w325) -> (error out=w323:errorcluster)  [unwired: 3 in, 5 out]
          n201 = local read "stopDolly"() -> (w321:bool)
          n202 = Compound Arithmetic op=OR(w321, w314, w306) -> (w316:bool)
          n203 = invoke on="3D Picture" class="SceneGraphDisp (strict)" method="Redraw"(error in=w323) -> ()  [unwired: 2 in, 3 out]
        }
        n204 = local write "drive"(w305) -> ()
      }
      frame "saveSetup" {
        n205 = Variant To Data(type=cluster{string, "appended path":path} {"", "appended path"=path ""} ("output cluster"), Variant=w332) -> (data=w331:cluster{string, "appended path":path})  [unwired: 1 in, 1 out]
        n206 = Unbundle(w331) -> (w329:string, "appended path"=w328:path)
        n207 = control-ref of="This VI"() -> (w334:refnum<vi>)
        n208 = call "INI-FP.vi"("Mode"=enum16{"Read", "Write"}."Write", "prompt"=w329, "VIreference"=w334, "INIfilepathIn"=w328) -> ("error out"=w327:errorcluster)  [unwired: 6 in, 1 out]
      }
      frame "stop" {
        n209 = call "3DplotterDataStore.vi"() -> ("3DplotterDataOut"=w350:T5)  [unwired: 11 in]
        n210 = Unbundle By Name(w350) -> ("refWorld"=w342:refnum<vi>, "refAxes"=w343:refnum<vi>, "refWindrose"=w344:refnum<vi>, "refGeometry"=w345:refnum<vi>, "geometryRefs"=w346:refnum<vi>[], "refVectors"=w347:refnum<vi>, "refVecs1"=w348:refnum<vi>, "refVecs2"=w349:refnum<vi>)
        n211 = Close Reference(reference=w349) -> (error out=w341:errorcluster)  [unwired: 1 in]
        n212 = Close Reference(reference=w348, error in (no error)=w341) -> (error out=w340:errorcluster)
        n213 = disable-structure shown="RUN_TIME_ENGINE==True" {
          frame condition #0 {
            n214 = control-ref of="This VI"() -> (w352:refnum<vi>)
            n215 = invoke class="VI" method="FP.Close"(reference=w352) -> ()  [unwired: 2 in, 3 out]
          }
          frame condition #1 (active) {
          }
        }
        n216 = Close Reference(reference=w347, error in (no error)=w340) -> (error out=w339:errorcluster)
        n217 = Close Reference(reference=w346, error in (no error)=w339) -> (error out=w338:errorcluster)
        n218 = Close Reference(reference=w345, error in (no error)=w338) -> (error out=w337:errorcluster)
        n219 = Close Reference(reference=w344, error in (no error)=w337) -> (error out=w336:errorcluster)
        n220 = Close Reference(reference=w343, error in (no error)=w336) -> (error out=w335:errorcluster)
        n221 = Close Reference(reference=w342, error in (no error)=w335) -> ()  [unwired: 1 out]
      }
    }
    "actionLoop" <- w10
    n222 = invoke on="3D Picture" class="SceneGraphDisp (strict)" method="Redraw"(error in=w10) -> ()  [unwired: 2 in, 3 out]
  }
  n223 = while {
    tunnel: w4 -> [w357]
    tunnel: w1 -> [w354]
    stop <- w356 stop-if-true
    n224 = event shown="[14] \"geometry\": Value Change" {
      selector: _ -> [_ _ _ _ _ _ _ _ _ _ _ _ _ _ _ _ _ _ _ _ _]
      dyn-events: _ -> [_ _ _ _ _ _ _ _ _ _ _ _ _ _ _ _ _ _ _ _ _]
      timeout: 1000 -> [_ _ _ _ _ _ _ _ _ _ _ _ _ _ _ _ _ _ _ _ _]
      tunnel: w357 -> [_ w361 _ w374 w376 w381 _ _ _ _ w414 w417 _ _ w427 w428 w430 w433 _ w455 w456]
      tunnel: [_ w360 _ _ _ _ _ _ _ _ _ _ _ _ _ _ _ _ _ _ _] -> w356
      tunnel: [_ _ _ _ _ _ _ _ _ _ _ _ _ _ _ _ w432 _ _ _ _] -> w355
      tunnel: w354 -> [_ w358 _ _ _ _ _ _ _ _ _ _ _ _ _ _ _ _ _ _ _]
      event Timeout {
        n225 = event-data() -> ()  [unwired: 1 in, 3 out]
      }
      event "Stop": Value Change {
        n226 = event-data() -> ()  [unwired: 1 in, 1 out]
        n227 = case shown="True" "Stop" {
          selector: "Stop" -> [w362 w371]
          tunnel: w361 -> [_ w370]
          tunnel: [w362 w371] -> w360
          tunnel: w358 -> [_ w368]
          frame False {
          }
          frame True {
            w363 = TRUE ("priority?")
            n228 = Bundle("", "appended path"=w368) -> (w367:cluster{string, "appended path":path})  [unwired: 1 in]
            n229 = call-poly "EnQ.vi"("priority?"=w363, "payload"=w367, "message"="saveSetup" ("String"), "EnQin"=w370) -> ("EnQout"=w365:refnum<queue>)  [unwired: 5 in, 2 out]
            n230 = call-poly "EnQ.vi"("priority?"=w363, "message"="stop", "EnQin"=w365) -> ()  [unwired: 6 in, 3 out]
          }
        }
        n231 = local write "stopDolly"(w360) -> ()
      }
      event Panel Close? {
        w372 = TRUE ("Value (Signaling)")
        n232 = event-data() -> ()  [unwired: 1 in, 1 out]
        n233 = property on="Stop" class="Bool"("Val(Sgnl)"=w372) -> ()  [unwired: 2 in, 2 out]
        n234 = event-data("Discard?"=w372) -> ()  [unwired: 1 in, 1 out]
      }
      event "vectorFile1", "vectorFile2": Value Change {
        n235 = event-data() -> ()  [unwired: 1 in, 4 out]
        n236 = call-poly "EnQ.vi"("messages"=string[] ["clearVectors", "loadFile1", "loadFile2"], "EnQin"=w374) -> ()  [unwired: 7 in, 3 out]
      }
      event "Vector Scale", "rampMin", "rampMax": Value Change {
        n237 = event-data() -> ()  [unwired: 1 in, 1 out]
        n238 = call-poly "EnQ.vi"("messages"=string[] ["clearVectors", "loadFile1", "loadFile2", "selectWD"], "EnQin"=w376) -> ()  [unwired: 7 in, 3 out]
      }
      event "axes": Value Change {
        n239 = event-data() -> ()  [unwired: 1 in, 1 out]
        n240 = Select(t="drawAxes" ("message"), s="axes", f="deleteAxes" ("message")) -> (s? t:f=w378:string)
        n241 = call-poly "EnQ.vi"("message"=w378, "EnQin"=w381) -> ()  [unwired: 7 in, 3 out]
      }
      event "axesColour": Value Change {
        n242 = event-data() -> ("NewVal"=w382:u32)  [unwired: 1 in, 5 out]
        n243 = call "3DplotterDataStore.vi"() -> ("3DplotterDataOut"=w386:T5)  [unwired: 11 in]
        n244 = Unbundle By Name(w386) -> ("refAxes"=w385:refnum<vi>)
        n245 = call <vilib>:"Color Change.vi"("Color"=w382) -> ("RGBA"=w383:cluster{"R":sgl, "G":sgl, "B":sgl, "A":sgl})  [unwired: 10 in]
        n246 = property class="SceneObject" props=["Material.Ambient", "Material.Color Mode", "Material.Diffuse", "Material.Emission", "Material.Shininess", "Material.Specular"](reference=w385, "Material.Ambient"=w383, "Material.Diffuse"=w383) -> (error out=w384:errorcluster)  [unwired: 1 in, 5 out]
        n247 = invoke on="3D Picture" class="SceneGraphDisp (strict)" method="Redraw"(error in=w384) -> ()  [unwired: 2 in, 3 out]
      }
      event "FoV", "depthClipping": Value Change {
        w389 = sgl 1000.0 ("y")
        # "Prevents inside-out world!"
        n248 = event-data() -> ()  [unwired: 1 in, 6 out]
        n249 = property on="3D Picture" class="SceneGraphDisp (strict)"() -> ("Content Bounds.Width"=w391:u32, "ContentBounds:Height"=w390:u32)  [unwired: 2 in, 2 out]
        n250 = Unbundle("depthClipping") -> (w394:sgl, w395:sgl)  [unwired: 1 out]
        n251 = Multiply(x=w394, y=w389) -> (x*y=w396:sgl)
        n252 = Multiply(x=w395, y=w389) -> (x*y=w397:sgl)
        n253 = Divide(x=w391, y=w390) -> (x/y=w392:dbl)
        n254 = Max & Min(x=w396, y=w397) -> (max(x,y)=w398:sgl, min(x,y)=w399:sgl)
        n255 = invoke on="3D Picture" class="SceneGraphDisp (strict)" method="Projection.Perspective"("Horizontal Field of View"="FoV", "Vertical Field of View"=w392, "Near Clipping Plane"=w399, "Far Clipping Plane"=w398) -> (error out=w393:errorcluster)  [unwired: 3 in, 6 out]
        n256 = invoke on="3D Picture" class="SceneGraphDisp (strict)" method="Redraw"(error in=w393) -> ()  [unwired: 2 in, 3 out]
      }
      event "3D Picture": Mouse Wheel {
        n257 = event-data() -> ("Delta"=w400:i32)  [unwired: 1 in, 9 out]
        n258 = local read "FoV"() -> (w401:sgl)
        n259 = Subtract(x=w401, y=w400) -> (x-y=w405:sgl)
        n260 = In Range and Coerce(upper limit=sgl 110.0, x=w405, lower limit=sgl 4.0) -> (coerced(x)=w404:sgl)  [unwired: 1 out]
        n261 = property on="FoV" class="Slide (strict)"("Val(Sgnl)"=w404) -> ()  [unwired: 2 in, 2 out]
      }
      event "3D Picture": Mouse Move {
        n262 = event-data() -> ()  [unwired: 1 in, 5 out]
        n263 = property on="3D Picture" class="SceneGraphDisp (strict)"() -> ("ModelView Matrix"=w408:sgl[][])  [unwired: 2 in, 2 out]
        n264 = call-poly <vilib>:"Inverse Matrix.vi"("matrix type"=T16."General", "Input Matrix"=w408) -> ("Inverse Matrix"=w412:T15)  [unwired: 1 out]
        n265 = call-poly <vilib>:"A x B.vi"("B"=T15 [[0.0], [0.0], [0.0], [1.0]], "A"=w412) -> ("A x B"=w410:T15)  [unwired: 1 out]
        n266 = Index Array(array=w410, index (col)=0 ("disabled index (col)")) -> (element=w406:dbl[])  [unwired: 1 in]
        n267 = property on="camLocn" class="Arr (strict)"("Val(Sgnl)"=w406) -> ()  [unwired: 2 in, 2 out]
      }
      event "clearVectors": Value Change {
        n268 = event-data() -> ()  [unwired: 1 in, 1 out]
        n269 = call-poly "EnQ.vi"("message"="clearVectors", "EnQin"=w414) -> ()  [unwired: 7 in, 3 out]
      }
      event "drive": Mouse Down {
        n270 = event-data() -> ()  [unwired: 1 in, 8 out]
        n271 = local write "stopDolly"(FALSE ("stopDolly")) -> ()
        n272 = call-poly "EnQ.vi"("message"="dollyMove", "EnQin"=w417) -> ()  [unwired: 7 in, 3 out]
      }
      event "drive": Mouse Up; "drive": Mouse Leave {
        n273 = event-data() -> ()  [unwired: 1 in, 4 out]
        "stopDolly" <- TRUE ("stopDolly")
      }
      event "camLocn": Value Change {
        n274 = event-data() -> ()  [unwired: 1 in, 1 out]
        n275 = call-poly <vilib>:"Dot Product.vi"("Y Vector"="camLocn", "X Vector"="camLocn") -> ("X * Y"=w425:dbl)  [unwired: 1 out]
        n276 = Square Root(x=w425) -> (sqrt(x)=w419:dbl)
        "camStandoff" <- w419
        n277 = Divide(x=w419, y=1000.0 ("x")) -> (x/y=w420:dbl)
        n278 = property on="depthClipping" class="Slide (strict)"() -> ("Value"=w423:cluster{sgl, sgl, sgl})  [unwired: 2 in, 2 out]
        n279 = Bundle(cluster=w423, w420) -> (w424:cluster{sgl, sgl, sgl})  [unwired: 2 in]
        n280 = property on="depthClipping" class="Slide (strict)"("Value"=w424) -> ()  [unwired: 2 in, 2 out]
      }
      event "geometry": Value Change {
        n281 = event-data() -> ()  [unwired: 1 in, 1 out]
        n282 = call-poly "EnQ.vi"("messages"=string[] ["clearGeometry", "loadGeometry", "buildGeometry", "renderGeometry", "geometrydZ"], "EnQin"=w427) -> ()  [unwired: 7 in, 3 out]
      }
      event "geometrydZ", "geometryScale": Value Change {
        n283 = event-data() -> ()  [unwired: 1 in, 1 out]
        n284 = call-poly "EnQ.vi"("message"="geometrydZ", "EnQin"=w428) -> ()  [unwired: 7 in, 3 out]
      }
      event "windrosePath", "Apply Mode", "windrosedXdYdZ", "windroseScale": Value Change {
        n285 = event-data() -> ()  [unwired: 1 in, 1 out]
        n286 = call-poly "EnQ.vi"("message"="renderWindrose", "EnQin"=w430) -> ()  [unwired: 7 in, 3 out]
        n287 = invoke on="3D Picture" class="SceneGraphDisp (strict)" method="Redraw"() -> (error out=w432:errorcluster)  [unwired: 3 in, 2 out]
      }
      event "Wind Direction Selector": Value Change; "view": Mouse Up {
        n288 = event-data() -> ()  [unwired: 1 in, 1 out]
        n289 = call-poly "EnQ.vi"("message"="selectWD", "EnQin"=w433) -> ()  [unwired: 7 in, 3 out]
      }
      event "3D Picture": Shortcut Menu Selection (User) {
        w438 = sgl 1000.0 ("y")
        n290 = event-data() -> ("CtlRef"=w446:refnum<vi>, "ItemTag"=w445:string)  [unwired: 1 in, 3 out]
        n291 = local read "depthClipping"() -> (w437:cluster{sgl, sgl, sgl})
        n292 = Unbundle(w437) -> (w439:sgl, w440:sgl)  [unwired: 1 out]
        n293 = local read "FoV"() -> (w443:sgl)
        n294 = Multiply(x=w439, y=w438) -> (x*y=w441:sgl)
        n295 = Multiply(x=w440, y=w438) -> (x*y=w442:sgl)
        n296 = Max & Min(x=w441, y=w442) -> (max(x,y)=w436:sgl, min(x,y)=w435:sgl)
        n297 = call "3DmenuHandler.vi"("nearClip"=w435, "farClip"=w436, "FoV"=w443, "ItemTag"=w445, "3DpicRef"=w446) -> ("error out"=w444:errorcluster)  [unwired: 6 in]
        n298 = invoke on="3D Picture" class="SceneGraphDisp (strict)" method="Redraw"(error in=w444) -> ()  [unwired: 2 in, 3 out]
      }
      event "exportSetup": Value Change {
        n299 = event-data() -> ()  [unwired: 1 in, 1 out]
        n300 = feedback #1() -> (w448:path)  [unwired: 1 in]
        n301 = Strip Path(path=w448) -> (stripped path=w449:path)  [unwired: 1 out]
        n302 = call "File Dialog"("start path"=w449, "pattern (all files)"="*.INI;*.ini", "pattern label"="Config Files") -> ("selected path"=w447:path)  [unwired: 9 in, 3 out]
        n303 = feedback-in #1(w447) -> ()
        n304 = Bundle("message"="Save 3-D Setup", "selected path"=w447) -> (w452:cluster{"message":string, "selected path":path})  [unwired: 1 in]
        n305 = call-poly "EnQ.vi"("payload"=w452, "message"="saveSetup", "EnQin"=w455) -> ()  [unwired: 6 in, 3 out]
      }
      event "importSetup": Value Change {
        n306 = event-data() -> ()  [unwired: 1 in, 1 out]
        n307 = Bundle("message"="Load 3-D Setup", path "") -> (w460:cluster{"message":string, path})  [unwired: 1 in]
        n308 = call-poly "EnQ.vi"("payload"=w460, "message"="init", "EnQin"=w456) -> ()  [unwired: 6 in, 3 out]
      }
    }
    "eventLoop" <- w355
  }
